vi "PID and FIT.vi"(0 "setpoint":dbl step=0.01 format="%.2f", 1 "X1(SetState)":T1(ring)=enum."max", 2 "reinitialize? (F)":bool, 5 "process variable":dbl step=0.01 format="%.2f", 7 "PID param":T2={"proportional gain (Kc)"=1.0, "integral time (Ti, s)"=10.0, "derivative time (Td, s)"=1.0, "output high"=100.0, "alr value"=0.0, "output low"=0.0, "output rate (EGU/s)"=1.0, "dt (s)"=-1.0} {"dt (s)" format="%.3f"; "output rate (EGU/s)" format="%.2f"; "output low" format="%.2f"; "alr value" format="%.2f"; "output high" format="%.2f"; "derivative time (Td, s)" format="%.3f"; "integral time (Ti, s)" format="%.3f"; "proportional gain (Kc)" format="%.3f"}, 9 "manual control":dbl format="%.2f", 12 "SP_massiv":dbl[](array[numeric])=[0.0, 10.0, 20.0, 30.0, 40.0, 50.0, 60.0, 70.0, 80.0, 90.0, 100.0] format="%#.2f", 13 "Y_massiv":dbl[](array[numeric])=[0.0, 0.0, 0.0, 0.0, 0.0, 0.0, 0.0, 0.0, 0.0, 0.0, 0.0] format="%#.2f", 14 "deadband":dbl=2.0 min=0.001 format="%.2f") -> (4 "output":dbl format="%.2f", 10 "dt out (s)":dbl format="%.3f")   [LabVIEW 2019, in "control.lvlib"]
uses:
  control.lvlib
  Inputs/Inputs.lvlib
panel:
  # "Входы\nX1(SetState) заданное состояние\n     0 – аварийное значение\n     1 – минимум\n     2 – стоп\n     3 – ручной\n     4 – автомат\n     5 – максимум"
  # "PID gains"
  # "output param"
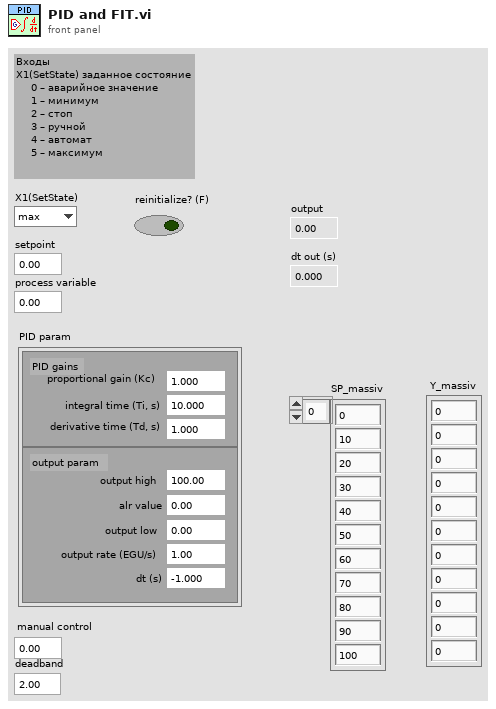
[diagram p1: front panel]
types:
  T1 = enum8{"alarm", "min", "stop", "hand", "auto", "max"}
  T2 = cluster{"proportional gain (Kc)":dbl, "integral time (Ti, s)":dbl, "derivative time (Td, s)":dbl, "output high":dbl, "alr value":dbl, "output low":dbl, "output rate (EGU/s)":dbl, "dt (s)":dbl}
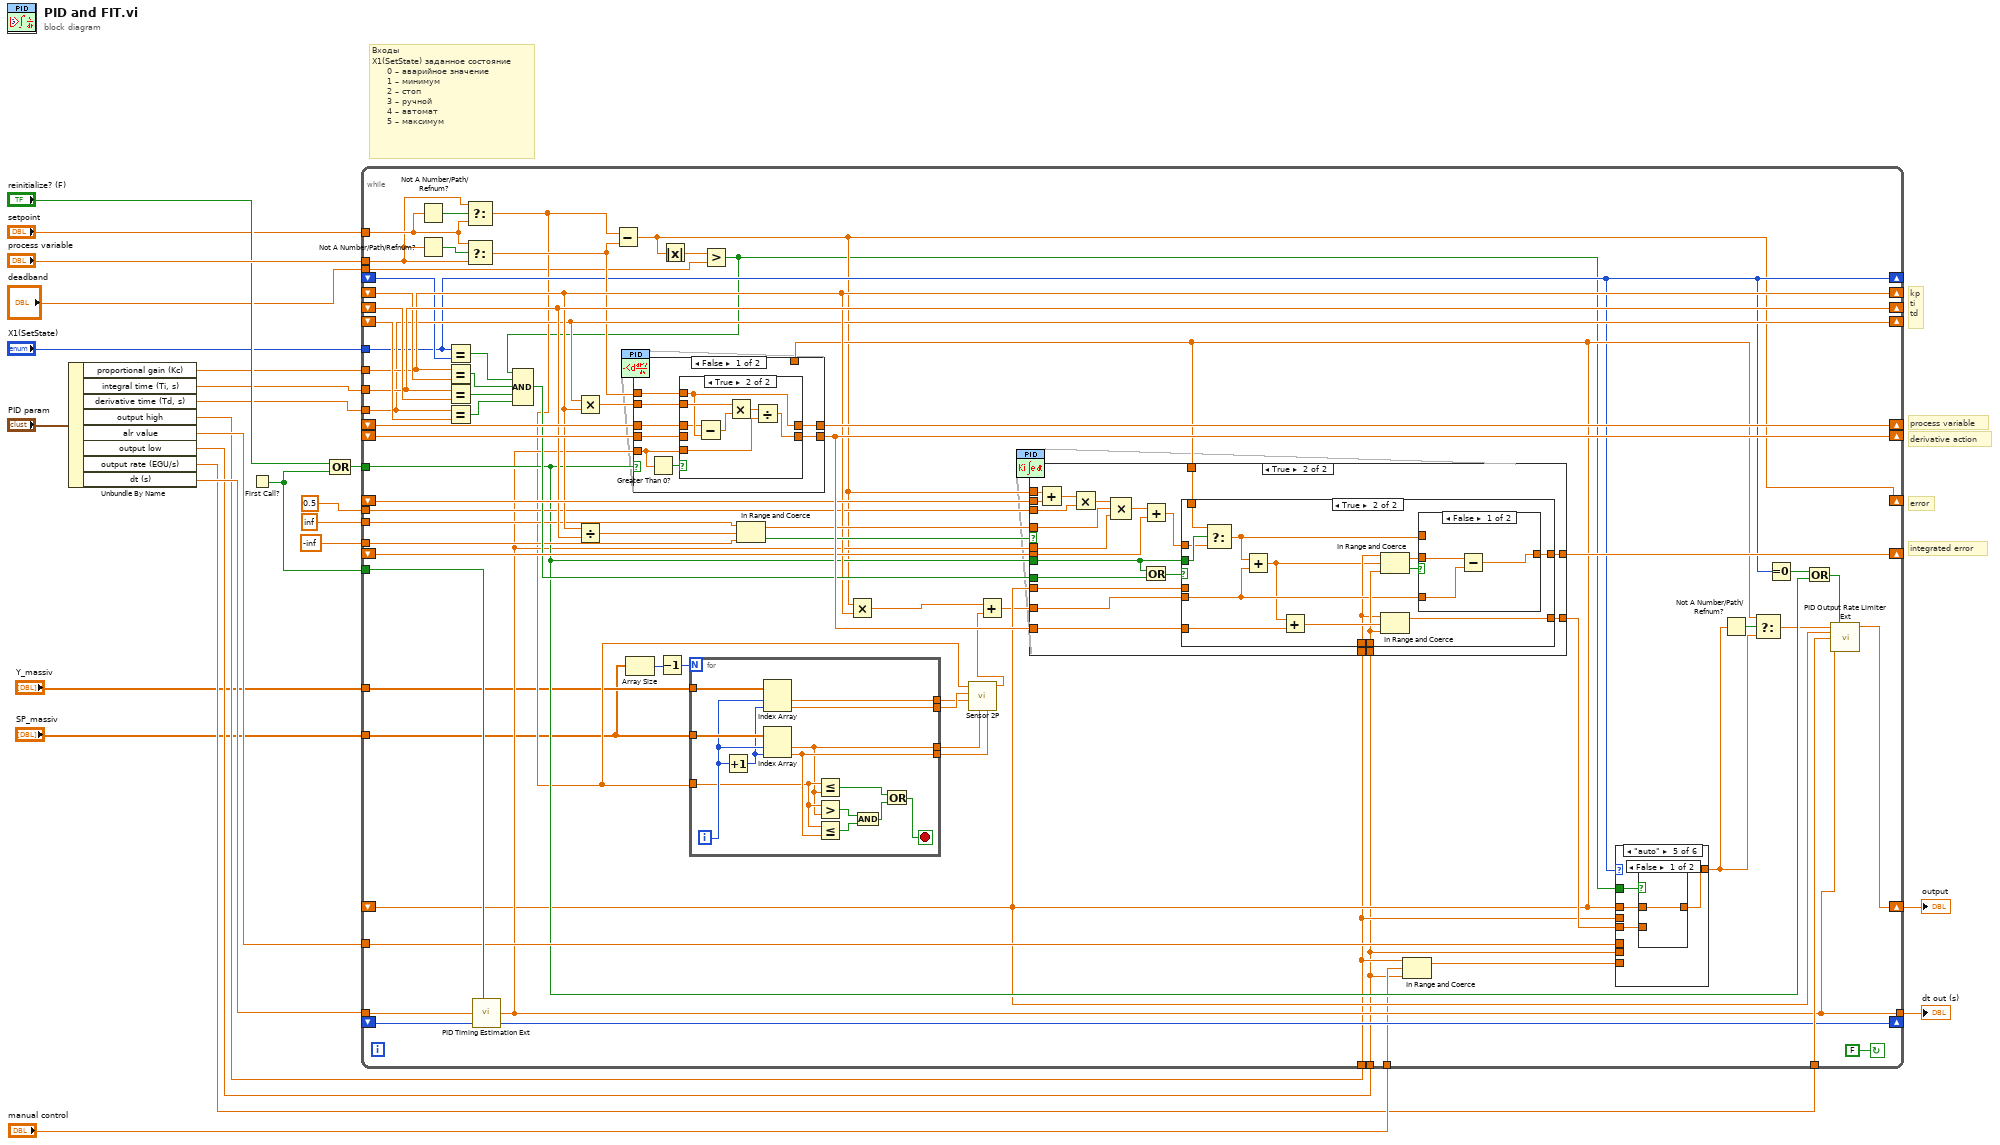
[diagram p0: block diagram]
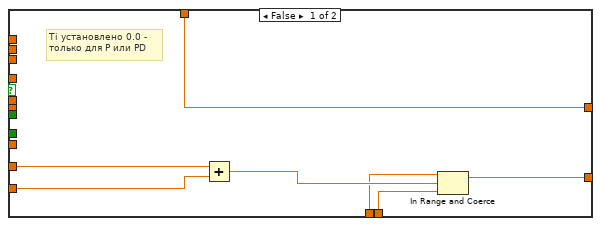
[diagram p2: hidden frame]
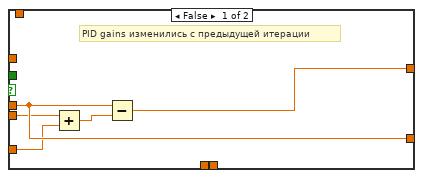
[diagram p3: hidden frame]
diagram:
  # "derivative action"
  # "process variable"
  # "kp\nti\ntd"
  # "error"
  # "integrated error"
  # "Входы\nX1(SetState) заданное состояние\n     0 – аварийное значение\n     1 – минимум\n     2 – стоп\n     3 – ручной\n     4 – автомат\n     5 – максимум"
  n1 = Unbundle By Name("PID param") -> ("proportional gain (Kc)"=w15:dbl, "integral time (Ti, s)"=w16:dbl, "derivative time (Td, s)"=w17:dbl, "output high"=w7:dbl, "alr value"=w9:dbl, "output low"=w6:dbl, "output rate (EGU/s)"=w5:dbl, "dt (s)"=w8:dbl)
  n2 = First Call?() -> (First Call?: T/F=w24:bool)
  n3 = Compound Arithmetic op=OR("reinitialize? (F)", w24) -> (w14:bool)
  n4 = while {
    tunnel: w14 -> [w52]
    shift-right: [w73] -> _
    shift-left: _ -> [w74]
    shift-right: [w75] -> _
    shift-left: _ -> [w92]
    shift-right: [w68] -> _
    shift-left: _ -> [w93]
    tunnel: w15 -> [w73]
    tunnel: w16 -> [w75]
    tunnel: w17 -> [w68]
    tunnel: w8 -> [w66]
    tunnel: w7 -> [w43]
    tunnel: w6 -> [w42]
    tunnel: "process variable" -> [w55]
    shift-right: [w88] -> _
    shift-left: _ -> [w87]
    shift-right: [w86] -> _
    shift-left: _ -> [w80]
    shift-right: [w28] -> _
    shift-left: _ -> [w85]
    shift-right: [w84] -> _
    shift-left: _ -> [w83]
    tunnel: 0.5 ("y") -> [w72]
    tunnel: inf ("upper limit") -> [w70]
    tunnel: -inf ("lower limit") -> [w71]
    tunnel: w24 -> [w67]
    tunnel: [w49] -> w13
    tunnel: "manual control" -> [w44]
    tunnel: w5 -> [w50]
    shift-right: [w53] -> w11
    shift-left: _ -> [w47]
    tunnel: w9 -> [w62]
    tunnel: "X1(SetState)" -> [w40]
    shift-right: [w40] -> _
    shift-left: _ -> [w61]
    tunnel: "setpoint" -> [w56]
    shift-right: [w46] -> _
    shift-left: _ -> [w45]
    tunnel: "Y_massiv" -> [w32]
    tunnel: "SP_massiv" -> [w29]
    tunnel: "deadband" -> [w26]
    stop <- FALSE continue-if-true
    n5 = Not A Number/Path/Refnum?(number/path/refnum=w56) -> (NaN/Path/Refnum?=w57:bool)
    n6 = Not A Number/Path/Refnum?(number/path/refnum=w55) -> (NaN/Path/Refnum?=w58:bool)
    n7 = Equal?(x=w40, y=w61) -> (x = y?=w60:bool)
    n8 = Equal?(x=w73, y=w74) -> (x = y?=w90:bool)
    n9 = Equal?(x=w75, y=w92) -> (x = y?=w89:bool)
    n10 = Equal?(x=w68, y=w93) -> (x = y?=w91:bool)
    n11 = Select(t=w55, s=w57, f=w56) -> (s? t:f=w33:dbl)
    n12 = Select(t=w56, s=w58, f=w55) -> (s? t:f=w59:dbl)
    n13 = call "PID Timing Estimation Ext.vi"("R"=w67, "dt (s) in"=w66, "Tick old"=w45) -> ("dt (s) out"=w49:dbl, "Tick"=w46:u32)  [unwired: 5 in]
    n14 = Multiply(x=w68, y=w73) -> (x*y=w79:dbl)
    n15 = Divide(x=w73, y=w75) -> (x/y=w78:dbl)
    n16 = Subtract(x=w33, y=w59) -> (x-y=w28:dbl)
    n17 = Array Size(array=w29) -> (size(s)=w38:i32)
    n18 = case shown="False" w52 {
      tunnel: w87 -> [w166 _]
      tunnel: w79 -> [w163 _]
      tunnel: w59 -> [w165 w177]
      tunnel: [w162 w177] -> w88
      tunnel: [w164 w176] -> w86
      tunnel: w80 -> [w160 _]
      tunnel: w49 -> [w159 _]
      tunnel: w47 -> [_ w176]
      frame False {
        n19 = Greater Than 0?(x=w159) -> (x > 0?=w161:bool)
        n20 = case shown="True" w161 {
          tunnel: w166 -> [w168 w169]
          tunnel: w159 -> [_ w174]
          tunnel: w165 -> [_ w170]
          tunnel: [w167 w173] -> w164
          tunnel: w163 -> [_ w172]
          tunnel: [w168 w170] -> w162
          tunnel: w160 -> [w167 _]
          frame False {
            # "dt = 0 min"
          }
          frame True {
            n21 = Subtract(x=w169, y=w170) -> (x-y=w171:dbl)
            n22 = Multiply(x=w172, y=w171) -> (x*y=w175:dbl)
            n23 = Divide(x=w175, y=w174) -> (x/y=w173:dbl)
          }
        }
      }
      frame True {
      }
    }
    n24 = Decrement(x=w38) -> (x-1=w39:i32)
    n25 = Absolute Value(x=w28) -> (abs(x)=w27:dbl)
    n26 = for {
      N: w39 -> [_]
      tunnel: w29 -> [w107]
      tunnel: w33 -> [w98]
      tunnel: [w97] -> w35
      tunnel: [w104] -> w34
      tunnel: w32 -> [w101]
      tunnel: [w100] -> w36
      tunnel: [w99] -> w37
      i -> [w103]
      stop <- w94 stop-if-true
      n27 = Increment(x=w103) -> (x+1=w102:i32)
      n28 = Index Array(array=w101, index #1=w103, index #2=w102) -> (element #1=w100:dbl, element #2=w99:dbl)
      n29 = Index Array(array=w107, index #1=w103, index #2=w102) -> (element #1=w97:dbl, element #2=w104:dbl)
      n30 = Less Or Equal?(x=w98, y=w97) -> (x <= y?=w95:bool)
      n31 = Greater?(x=w98, y=w97) -> (0:w106:bool)
      n32 = Less Or Equal?(x=w98, y=w104) -> (x <= y?=w105:bool)
      n33 = And(x=w106, y=w105) -> (x .and. y?=w96:bool)
      n34 = Or(x=w95, y=w96) -> (x .or. y?=w94:bool)
    }
    n35 = Greater?(x=w27, y=w26) -> (0:w25:bool)
    n36 = Compound Arithmetic op=AND(w25, w60, w90, w89, w91) -> (w76:bool)
    n37 = In Range and Coerce(upper limit=w70, x=w78, lower limit=w71) -> (coerced(x)=w82:dbl, In Range?=w81:bool)
    n38 = Multiply(x=w28, y=w73) -> (x*y=w77:dbl)
    n39 = call "Sensor 2P.vi"("Xmax"=w34, "Xmin"=w35, "Ymin"=w36, "Ymax"=w37, "X"=w33) -> ("Y"=w30:dbl)  [unwired: 6 in]
    n40 = Add(x=w77, y=w30) -> (x+y=w31:dbl)
    n41 = case shown="True" w81 {
      tunnel: w28 -> [_ w134]
      tunnel: w85 -> [_ w135]
      tunnel: w83 -> [_ w130]
      tunnel: [w108 w125] -> w84
      tunnel: w82 -> [_ w123]
      tunnel: w31 -> [w113 w128]
      tunnel: [w114 w124] -> w64
      tunnel: w47 -> [_ w126]
      tunnel: w86 -> [w112 w122]
      tunnel: w52 -> [_ w121]
      tunnel: w76 -> [_ w120]
      tunnel: w49 -> [_ w119]
      tunnel: w43 -> [w110 w117]
      tunnel: w42 -> [w109 w118]
      tunnel: w72 -> [_ w116]
      tunnel: w47 -> [w108 w115]
      frame False {
        # "Ti установлено 0.0 -\nтолько для P или PD"
        n42 = Add(x=w113, y=w112) -> (x+y=w111:dbl)
        n43 = In Range and Coerce(upper limit=w110, x=w111, lower limit=w109) -> (coerced(x)=w114:dbl)  [unwired: 1 out]
      }
      frame True {
        n44 = Add(x=w134, y=w135) -> (x+y=w133:dbl)
        n45 = Multiply(x=w133, y=w116) -> (x*y=w132:dbl)
        n46 = Compound Arithmetic op=MULTIPLY(w132, w123, w119) -> (w131:dbl)
        n47 = Add(x=w131, y=w130) -> (x+y=w129:dbl)
        n48 = Or(x=w121, y=w120) -> (x .or. y?=w127:bool)
        n49 = case shown="True" w127 {
          tunnel: w129 -> [_ w141]
          tunnel: w128 -> [w138 w147]
          tunnel: w126 -> [w140 _]
          tunnel: w121 -> [_ w144]
          tunnel: [w139 w149] -> w125
          tunnel: [w140 w153] -> w124
          tunnel: w122 -> [w137 w152]
          tunnel: w118 -> [_ w151]
          tunnel: w117 -> [_ w146]
          tunnel: w115 -> [_ w143]
          frame False {
            # "PID gains изменились с предыдущей итерации"
            n50 = Add(x=w138, y=w137) -> (x+y=w136:dbl)
            n51 = Subtract(x=w140, y=w136) -> (x-y=w139:dbl)
          }
          frame True {
            n52 = Select(t=w143, s=w144, f=w141) -> (s? t:f=w142:dbl)
            n53 = Add(x=w142, y=w147) -> (x+y=w145:dbl)
            n54 = Add(x=w145, y=w152) -> (x+y=w154:dbl)
            n55 = In Range and Coerce(upper limit=w146, x=w145, lower limit=w151) -> (coerced(x)=w148:dbl, In Range?=w150:bool)
            n56 = In Range and Coerce(upper limit=w146, x=w154, lower limit=w151) -> (coerced(x)=w153:dbl)  [unwired: 1 out]
            n57 = case shown="False" w150 {
              tunnel: w142 -> [_ w158]
              tunnel: [w155 w158] -> w149
              tunnel: w148 -> [w157 _]
              tunnel: w147 -> [w156 _]
              frame False {
                n58 = Subtract(x=w157, y=w156) -> (x-y=w155:dbl)
              }
              frame True {
              }
            }
          }
        }
      }
    }
    n59 = In Range and Coerce(upper limit=w43, x=w44, lower limit=w42) -> (coerced(x)=w41:dbl)  [unwired: 1 out]
    n60 = case shown="\"auto\"" w40 {
      tunnel: w47 -> [_ _ w180 _ w182 _]
      tunnel: w64 -> [_ _ _ _ w184 _]
      tunnel: w41 -> [_ _ _ w181 _ _]
      tunnel: [w178 w179 w180 w181 w183 w188] -> w63
      tunnel: w62 -> [w178 _ _ _ _ _]
      tunnel: w43 -> [_ _ _ _ _ w188]
      tunnel: w42 -> [_ w179 _ _ _ _]
      tunnel: w25 -> [_ _ _ _ w185 _]
      frame "alarm", Default {
      }
      frame "min" {
      }
      frame "stop" {
      }
      frame "hand" {
      }
      frame "auto" {
        n61 = case shown="False" w185 {
          tunnel: w184 -> [_ w187]
          tunnel: [w186 w187] -> w183
          tunnel: w182 -> [w186 _]
          frame False {
          }
          frame True {
          }
        }
      }
      frame "max" {
      }
    }
    n62 = Not A Number/Path/Refnum?(number/path/refnum=w63) -> (NaN/Path/Refnum?=w65:bool)
    n63 = Select(t=w47, s=w65, f=w63) -> (s? t:f=w48:dbl)
    n64 = Equal To 0?(x=w40) -> (x = 0?=w54:bool)
    n65 = Or(x=w54, y=w52) -> (x .or. y?=w51:bool)
    n66 = call "PID Output Rate Limiter Ext.vi"("input (controller output)"=w48, "reinitialize? (F)"=w51, "output old"=w47, "output rate (EGU/s)"=w50, "dt (s)"=w49) -> ("output"=w53:dbl)  [unwired: 8 in, 2 out]
  }
  "output" <- w11
  "dt out (s)" <- w13
